vi "Main LIEF 3.vi"() -> ()   [LabVIEW 2015]
uses:
  <vilib>/LIEF/Image Editor Handler/Image Editor Handler.lvclass
  <vilib>/LIEF/Forms/Rectangle/Rectangle.lvclass
  <vilib>/LIEF/Forms/Shape/Shape.lvclass/Shape.ctl
  <vilib>/LIEF/Forms/Rectangle/Rectangle.lvclass/Rectangle.ctl
  <vilib>/LIEF/Forms/Layered Shape/Layered Shape.lvclass/Layered Shape.ctl
  <vilib>/LIEF/Forms/Shape/Write Color.vi
  <vilib>/LIEF/Forms/Rectangle/Write Filled.vi
  <vilib>/LIEF/Forms/Layered Shape/Write Overlays.vi
  <vilib>/LIEF/Forms/Shape/Shape.lvclass
  <vilib>/LIEF/Forms/Text/Text.lvclass
panel:
  in  "2D Picture":picture
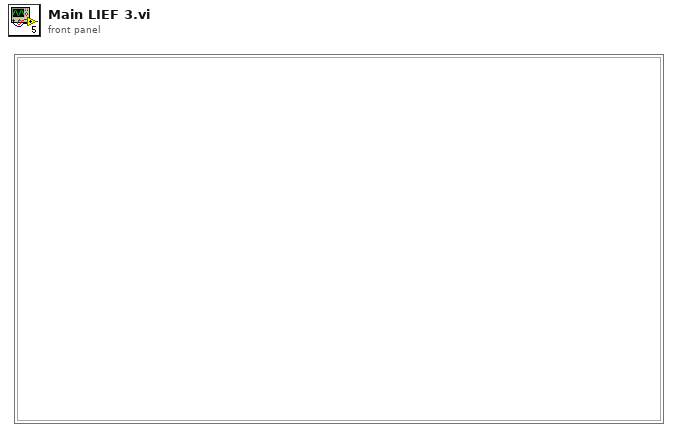
[diagram p1: front panel]
types:
  T1 = enum16{"Left", "Top", "Right", "Bottom", "Centered"}
  T2 = cluster{"Font Name:":string, "Size":i16, "Strikeout?":bool, "Italic?":bool, "Underline?":bool, "Outline?":bool, "Shadow?":bool, "Bold?":bool}
  T3 = cluster{"Block Name":string, "Inputs":string[], "Outputs":string[]}
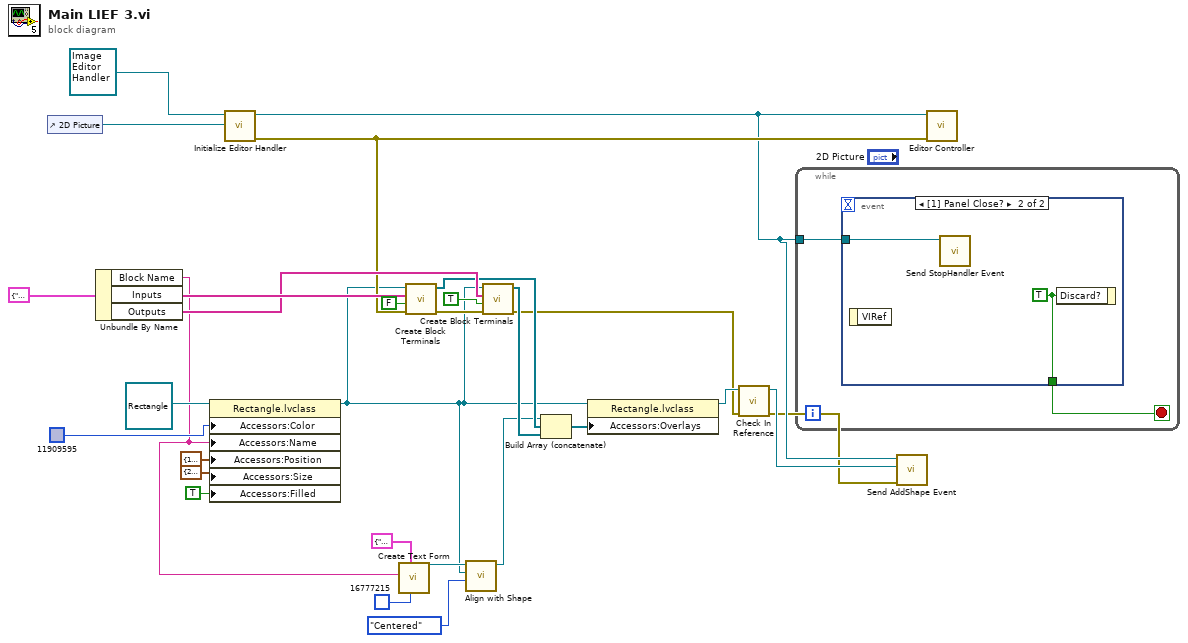
[diagram p0: block diagram]
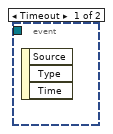
[diagram p2: hidden frame]
diagram:
  n1 = control-ref of="2D Picture"() -> (w28:refnum<vi>)
  n2 = Unbundle By Name(T3 {"Block Name"="Generator", "Inputs"=["Freq", "Gain"], "Outputs"=["Amplitude", "Phase", "Error"]}) -> ("Block Name"=w7:string, "Inputs"=w26:string[], "Outputs"=w18:string[])
  n3 = property class="Rectangle.lvclass"(reference=refnum<class "Rectangle.lvclass"> refnum ("Rectangle in"), "Accessors:Color"=u32 11909595, "Accessors:Name"=w7, "Accessors:Position"=cluster{"Left":i32, "Top":i32} {"Left"=100, "Top"=100} ("Position"), "Accessors:Size"=cluster{"Width":i32, "Height":i32} {"Width"=200, "Height"=160} ("Size"), "Accessors:Filled"=TRUE ("Filled")) -> (reference out=w3:refnum<class "Rectangle.lvclass">)  [unwired: 1 in, 1 out]
  n4 = call <vilib>:"Initialize Editor Handler.vi"("PictureRef"=w28, "Editor Handler in"=refnum<class "Image Editor Handler.lvclass"> refnum) -> ("error out"=w14:errorcluster, "Editor Handler out"=w10:refnum<class "Image Editor Handler.lvclass">)  [unwired: 8 in]
  n5 = call <vilib>:"Create Text Form.vi"("Color"=u32 16777215, "[user-specified font]"=T2 {"Font Name:"="Segoe UI", "Size"=18, "Strikeout?"=FALSE, "Italic?"=FALSE, "Underline?"=FALSE, "Outline?"=FALSE, "Shadow?"=FALSE, "Bold?"=TRUE}, "Text"=w7) -> ("New Text"=w4:refnum<class "Text.lvclass">)  [unwired: 7 in, 1 out]
  n6 = call "Create Block Terminals.vi"("error in (no error)"=w14, "Output?"=FALSE ("Direction"), "Inputs"=w26, "Rectangle in"=w3) -> ("error out"=w13:errorcluster, "Array"=w17:refnum<class "Terminal.lvclass">[])  [unwired: 6 in]
  n7 = call <vilib>:"Align with Shape.vi"("Alignment"=T1."Centered", "Reference Shape"=w3, "Shape in"=w4) -> ("Shape out"=w1:refnum<class "Text.lvclass">)  [unwired: 7 in, 1 out]
  n8 = call "Create Block Terminals.vi"("error in (no error)"=w13, "Output?"=TRUE ("Direction"), "Inputs"=w18, "Rectangle in"=w3) -> ("error out"=w8:errorcluster, "Array"=w16:refnum<class "Terminal.lvclass">[])  [unwired: 6 in]
  n9 = Build Array (concatenate)(w1, w17, w16) -> (w15:refnum<class "Shape.lvclass">[])
  n10 = property class="Rectangle.lvclass"(reference=w3, "Accessors:Overlays"=w15) -> (reference out=w12:refnum<class "Rectangle.lvclass">)  [unwired: 1 in, 1 out]
  n11 = call <vilib>:"Check In Reference.vi"("error in (no error)"=w8, "Shape in"=w12) -> ("error out"=w9:errorcluster, "Shape Reference"=w11:refnum<data-value>)  [unwired: 8 in]
  n12 = while {
    tunnel: w10 -> [w30]
    stop <- w31 stop-if-true
    n13 = event shown="[1] Panel Close?" {
      selector: _ -> [_ _]
      dyn-events: _ -> [_ _]
      timeout: _ -> [_ _]
      tunnel: [_ w33] -> w31
      tunnel: w30 -> [_ w32]
      event Timeout {
        n14 = event-data() -> ()  [unwired: 1 in, 3 out]
      }
      event Panel Close? {
        w33 = TRUE ("Discard?")
        n15 = event-data() -> ()  [unwired: 1 in, 1 out]
        n16 = call <vilib>:"Send StopHandler Event.vi"("Editor Handler in"=w32) -> ()  [unwired: 9 in, 2 out]
        n17 = event-data("Discard?"=w33) -> ()  [unwired: 1 in, 1 out]
      }
    }
  }
  n18 = call <vilib>:"Send AddShape Event.vi"("error in (no error)"=w9, "New Shape Reference"=w11, "Editor Handler in"=w10) -> ()  [unwired: 7 in, 2 out]
  n19 = call <vilib>:"Editor Controller.vi"("error in (no error)"=w14, "Editor Handler in"=w10) -> ()  [unwired: 8 in, 2 out]
